vi "Draw Zones on Field.vi"(10 "Zones In":T1[](array[typedef]), 11 "new picture in":picture) -> (3 "new picture out":picture)   [LabVIEW 2015]
uses:
  Typedef/Zone Data.ctl
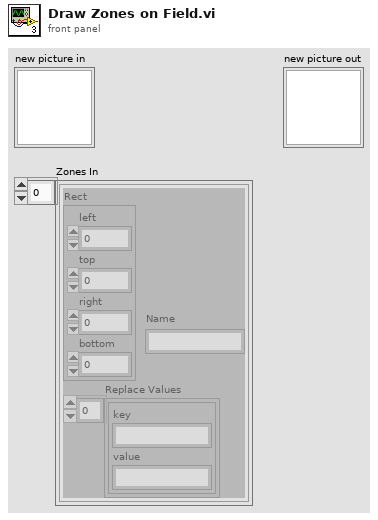
[diagram p1: front panel]
types:
  T1 = typedef "Zone Data.ctl" = cluster{"Rect":cluster{"left":i16, "top":i16, "right":i16, "bottom":i16}, "Replace Values":cluster{"key":string, "value":string}[], "Name":string}
  T2 = cluster{"left":i16, "top":i16, "right":i16, "bottom":i16}
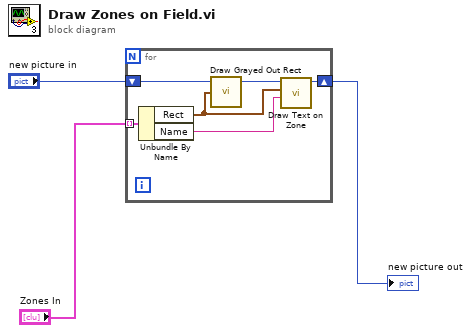
[diagram p0: block diagram]
diagram:
  n1 = for {
    shift-right: [w6] -> w2
    shift-left: "new picture in" -> [w8]
    tunnel: "Zones In" -> [w9] mode=indexing
    n2 = Unbundle By Name(w9) -> ("Rect"=w4:T2, "Name"=w5:string)
    n3 = call <vilib>:"Draw Grayed Out Rect.vi"("rect"=w4, "picture"=w8) -> ("new picture"=w7:picture)  [unwired: 3 in]
    n4 = call "Draw Text on Zone.vi"("Name"=w5, "rect"=w4, "Field"=w7) -> ("new picture"=w6:picture)  [unwired: 8 in]
  }
  "new picture out" <- w2
